vi "NI-Sync_test_case.vi"() -> ()   [LabVIEW 2015]
uses:
  <vilib>/userdefined/High Color/nirio_resource_hc.ctl
  <vilib>/DAQmx/read.llb/DAQmx Read (Analog Wfm 1Chan NSamp).vi
  <instrlib>/niSync/niSync.llb/niSync Initialize (IVI).vi
  <vilib>/DAQmx/create/channels.llb/DAQmx Create Channel (AI-Voltage-Basic).vi
  <vilib>/DAQmx/configure/timing.llb/DAQmx Timing (Sample Clock).vi
  <vilib>/DAQmx/create/channels.llb/DAQmx Create Channel (CO-Pulse Generation-Time).vi
  <vilib>/DAQmx/configure/timing.llb/DAQmx Timing (Implicit).vi
  <vilib>/DAQmx/configure/trigger.llb/DAQmx Start Trigger (Digital Edge).vi
  <vilib>/DAQmx/miscellaneous.llb/DAQmx Fill In Error Info.vi
  <vilib>/FPGAPlugInAG/Dynamic/niLvFpga_Close_Dynamic.vi
  <vilib>/rvi/interface/nirviCloseFPGA/nirviCloseFPGA.xnode
  <resource>/objmgr/daqmx.rc
panel:
  in  "Reset sync cards?":bool
  in  "Pulse delay":dbl=0.0001 format="%#_13g"
  in  "Pulse counter destination terminal":string(combo)="PXI_Star1"
  in  "DAQ pulse gen looking at:":tag="/Timing1/PXI_Star"
  in  "DAQ pulse gen counter":tag="Timing1/ctr2"
  in  "DAQ Physical Channel":tag="DAQ0/ai3"
  in  "Num samples: DAQ":i32=1000
  in  "FPGA AI to plot":i32
  out "RIO":waveform(dbl)(graph)
  out "Interleaved Raw Data":u64[](array[numeric])
  out "Counts":i16[][](array[numeric])
  out "Voltage":dbl[][](array[numeric])
  in  "FPGA delay (x 50ns)":u64=2
  in  "Num samples: RIO":u64=20000
  in  "FPGA name":T1="RIO0" caption="RIO Device"
  out "DAQ":waveform(dbl)(graph)
  in  "DAQ listens to":tag="/DAQ0/PXI_Star"
  in  "DAQ Delay (s)":dbl=1e-07
  in  "RIO Destination Terminal":string(combo)="PXI_Star0"
  in  "DAQ destination terminal":string(combo)="PXI_Star2"
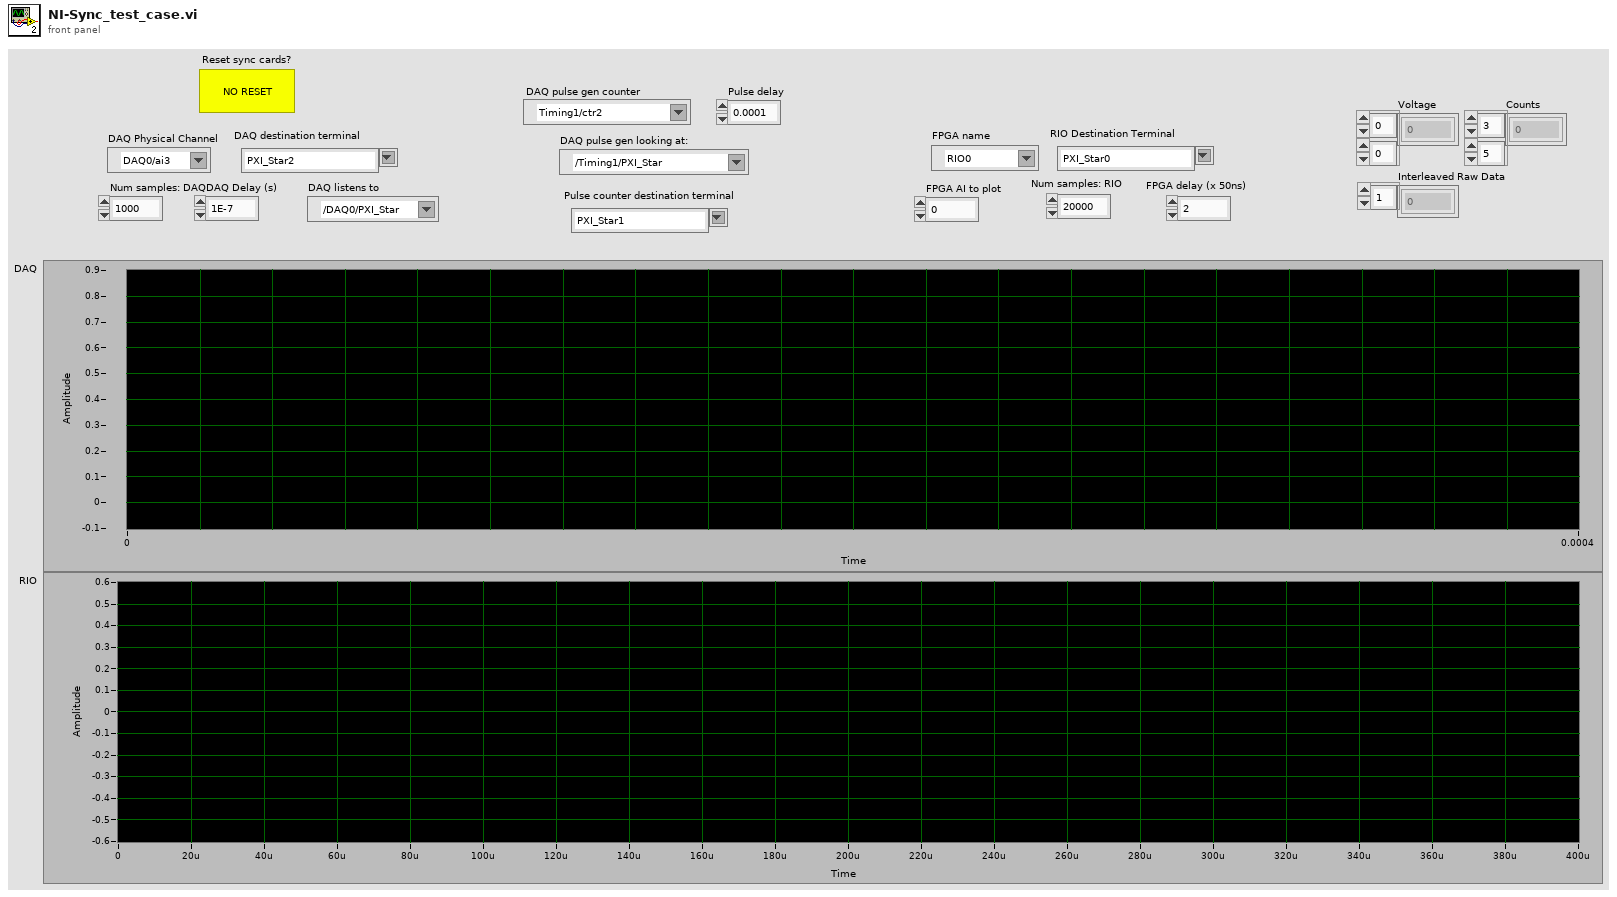
[diagram p1: front panel]
types:
  T1 = typedef "nirio_resource_hc.ctl" = tag
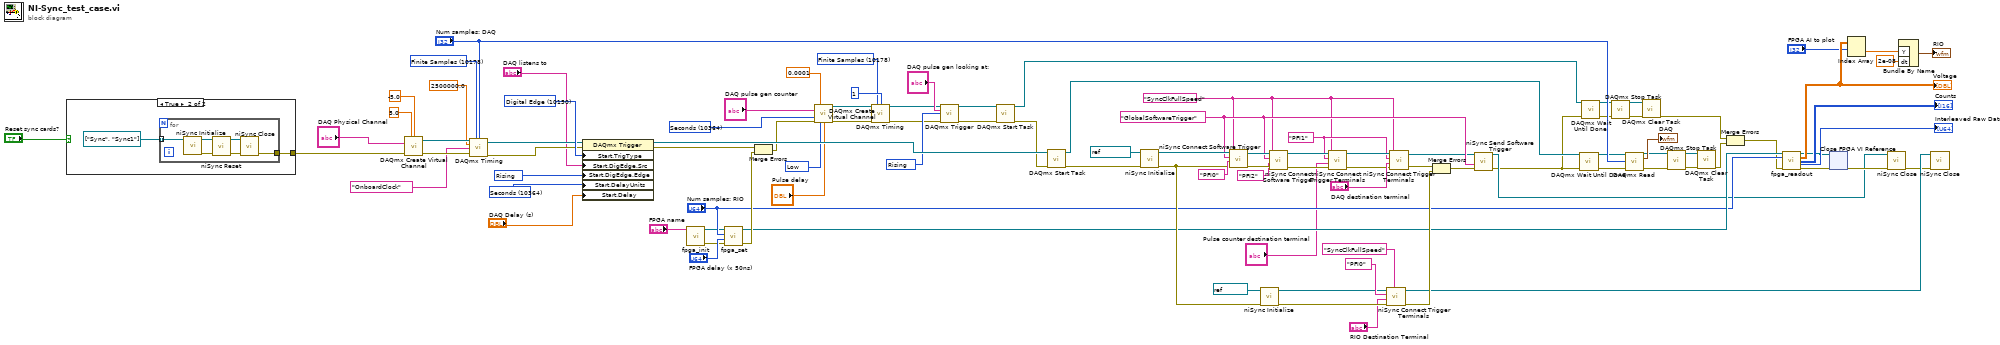
[diagram p0: block diagram]
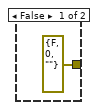
[diagram p2: hidden frame]
diagram:
  w24 = 10178 items=["Finite Samples"=10178, "Continuous Samples"=10123, "Hardware Timed Single Point"=12522] ("sample mode")
  w30 = 10280 items=["Rising"=10280, "Falling"=10171] ("edge")
  w32 = 10364 items=["Seconds"=10364] ("units")
  w33 = 10214 items=["High"=10192, "Low"=10214] ("idle state")
  w66 = 10280 items=["Rising"=10280, "Falling"=10171] ("Start.DigEdge.Edge")
  w71 = 10364 items=["Sample Clock Periods"=10286, "Seconds"=10364, "Ticks"=10304] ("Start.DelayUnits")
  w72 = 10150 items=["Analog Edge"=10099, "Digital Edge"=10150, "Digital Pattern"=10398, "Analog Window"=10103, "None"=10230] ("Start.TrigType")
  w74 = 10178 items=["Finite Samples"=10178, "Continuous Samples"=10123, "Hardware Timed Single Point"=12522] ("sample mode")
  w7 = "PFI1" ("source terminal")
  w6 = "SyncClkFullSpeed" ("synchronization clock")
  w85 = "GlobalSoftwareTrigger" ("source terminal")
  n1 = case shown="True" "Reset sync cards?" {
    tunnel: [errorcluster {"status"=FALSE, "code"=0, "source"=""} ("error out") w103] -> w2
    frame False {
    }
    frame True {
      n2 = for {
        tunnel: refnum<k15>[] ["Sync", "Sync1"] -> [w108] mode=indexing
        tunnel: [w105] -> w103
        n3 = call-poly <instrlib>:"niSync Initialize.vi"("resource name"=w108) -> ("error out"=w109:errorcluster, "instrument handle out"=w110:refnum<k15>)  [unwired: 9 in]
        n4 = call <instrlib>:"niSync Reset.vi"("error in (no error)"=w109, "instrument handle"=w110) -> ("error out"=w106:errorcluster, "instrument handle out"=w107:refnum<k15>)  [unwired: 8 in]
        n5 = call <instrlib>:"niSync Close.vi"("error in (no error)"=w106, "instrument handle"=w107) -> ("error out"=w105:errorcluster)  [unwired: 9 out]
      }
    }
  }
  n6 = call-poly <vilib>:"DAQmx Create Virtual Channel.vi"("maximum value"=5.0, "minimum value"=-5.0, "physical channels"="DAQ Physical Channel", "error in"=w2) -> ("task out"=w78:refnum<k21>, "error out"=w77:errorcluster)  [unwired: 10 in]
  n7 = call-poly <vilib>:"DAQmx Timing.vi"("task/channels in"=w78, "sample mode"=w74, "samples per channel"="Num samples: DAQ", "rate"=2500000.0, "source"=tag "OnboardClock", "error in"=w77) -> ("task out"=w69:refnum<k21>, "error out"=w68:errorcluster)  [unwired: 8 in]
  n8 = property class="DAQmx Trigger"(reference=w69, error in=w68, "Start.TrigType"=w72, "Start.DigEdge.Src"="DAQ listens to", "Start.DigEdge.Edge"=w66, "Start.DelayUnits"=w71, "Start.Delay"="DAQ Delay (s)") -> (reference out=w64:refnum<k21>, error out=w46:errorcluster)
  n9 = call "fpga_init.vi"("FPGA name"="FPGA name") -> ("error out"=w3:errorcluster, "FPGA VI Reference Out"=w4:refnum<k20>)  [unwired: 9 in]
  n10 = call "fpga_set.vi"("error in"=w3, "trigger  delay"="FPGA delay (x 50ns)", "num samples"="Num samples: RIO", "FPGA VI Reference In"=w4) -> ("error out"=w45:errorcluster, "FPGA VI Reference Out"=w43:refnum<k20>)  [unwired: 6 in]
  n11 = Merge Errors(w46, w45) -> (w36:errorcluster)
  n12 = call-poly <vilib>:"DAQmx Create Virtual Channel.vi"("high time"=0.0001, "counter"="DAQ pulse gen counter", "units"=w32, "error in"=w36, "idle state"=w33, "initial delay"="Pulse delay") -> ("task out"=w29:refnum<k21>, "error out"=w27:errorcluster)  [unwired: 8 in]
  n13 = call-poly <vilib>:"DAQmx Timing.vi"("task/channels in"=w29, "sample mode"=w24, "samples per channel"=1, "error in"=w27) -> ("task out"=w28:refnum<k21>, "error out"=w26:errorcluster)  [unwired: 10 in]
  n14 = call-poly <vilib>:"DAQmx Trigger.vi"("task/channels in"=w28, "source"="DAQ pulse gen looking at:", "edge"=w30, "error in"=w26) -> ("task out"=w21:refnum<k21>, "error out"=w23:errorcluster)  [unwired: 10 in]
  n15 = call <vilib>:"DAQmx Start Task.vi"("task/channels in"=w21, "error in"=w23) -> ("task out"=w16:refnum<k21>, "error out"=w22:errorcluster)  [unwired: 12 in]
  n16 = call <vilib>:"DAQmx Start Task.vi"("task/channels in"=w64, "error in"=w22) -> ("task out"=w39:refnum<k21>, "error out"=w65:errorcluster)  [unwired: 12 in]
  n17 = call-poly <instrlib>:"niSync Initialize.vi"("error in (no error)"=w65, "resource name"=refnum<k15> "Sync") -> ("error out"=w73:errorcluster, "instrument handle out"=w99:refnum<k15>)  [unwired: 1 in, 7 out]
  n18 = call <instrlib>:"niSync Connect Software Trigger.vi"("synchronization clock"=w6, "error in (no error)"=w73, "destination terminal"="PFI0", "source terminal"=w85, "instrument handle"=w99) -> ("error out"=w96:errorcluster, "instrument handle out"=w97:refnum<k15>)  [unwired: 2 in, 3 out]
  n19 = call-poly <instrlib>:"niSync Initialize.vi"("error in (no error)"=w73, "resource name"=refnum<k15> "Sync1") -> ("error out"=w94:errorcluster, "instrument handle out"=w90:refnum<k15>)  [unwired: 1 in, 7 out]
  n20 = call <instrlib>:"niSync Connect Software Trigger.vi"("synchronization clock"=w6, "error in (no error)"=w96, "destination terminal"="PFI2", "source terminal"=w85, "instrument handle"=w97) -> ("error out"=w9:errorcluster, "instrument handle out"=w11:refnum<k15>)  [unwired: 2 in, 3 out]
  n21 = call <instrlib>:"niSync Connect Trigger Terminals.vi"("synchronization clock"=w6, "error in (no error)"=w9, "destination terminal"="Pulse counter destination terminal", "source terminal"=w7, "instrument handle"=w11) -> ("error out"=w8:errorcluster, "instrument handle out"=w10:refnum<k15>)  [unwired: 5 in]
  n22 = call <instrlib>:"niSync Connect Trigger Terminals.vi"("synchronization clock"="SyncClkFullSpeed", "error in (no error)"=w94, "destination terminal"="RIO Destination Terminal", "source terminal"="PFI0", "instrument handle"=w90) -> ("error out"=w91:errorcluster, "instrument handle out"=w83:refnum<k15>)  [unwired: 5 in]
  n23 = call <instrlib>:"niSync Connect Trigger Terminals.vi"("synchronization clock"=w6, "error in (no error)"=w8, "destination terminal"="DAQ destination terminal", "source terminal"=w7, "instrument handle"=w10) -> ("error out"=w89:errorcluster, "instrument handle out"=w84:refnum<k15>)  [unwired: 5 in]
  n24 = Merge Errors(w89, w91) -> (w86:errorcluster)
  n25 = call <instrlib>:"niSync Send Software Trigger.vi"("error in (no error)"=w86, "source terminal"=w85, "instrument handle"=w84) -> ("error out"=w15:errorcluster, "instrument handle out"=w41:refnum<k15>)  [unwired: 7 out]
  n26 = call <vilib>:"DAQmx Wait Until Done.vi"("task/channels in"=w39, "error in"=w15) -> ("task out"=w40:refnum<k21>, "error out"=w38:errorcluster)  [unwired: 12 in]
  n27 = call <vilib>:"DAQmx Wait Until Done.vi"("task/channels in"=w16, "error in"=w15) -> ("task out"=w18:refnum<k21>, "error out"=w17:errorcluster)  [unwired: 12 in]
  n28 = call <vilib>:"DAQmx Stop Task.vi"("task/channels in"=w18, "error in"=w17) -> ("task out"=w19:refnum<k21>, "error out"=w20:errorcluster)  [unwired: 12 in]
  n29 = call-poly <vilib>:"DAQmx Read.vi"("task/channels in"=w40, "number of samples per channel"="Num samples: DAQ", "error in"=w38) -> ("task out"=w61:refnum<k21>, "data"=→"DAQ":waveform(dbl), "error out"=w62:errorcluster)  [unwired: 10 in]
  n30 = call <vilib>:"DAQmx Clear Task.vi"("task in"=w19, "error in"=w20) -> ("error out"=w14:errorcluster)  [unwired: 13 in]
  n31 = call <vilib>:"DAQmx Stop Task.vi"("task/channels in"=w61, "error in"=w62) -> ("task out"=w59:refnum<k21>, "error out"=w58:errorcluster)  [unwired: 12 in]
  n32 = call <vilib>:"DAQmx Clear Task.vi"("task in"=w59, "error in"=w58) -> ("error out"=w13:errorcluster)  [unwired: 13 in]
  n33 = Merge Errors(w14, w13) -> (w12:errorcluster)
  n34 = call "fpga_readout.vi"("FPGA VI Reference In"=w43, "samples"="Num samples: RIO", "error in"=w12) -> ("FPGA Reference Out"=w44:refnum<k20>, "Voltage"=w49:dbl[][], "Counts"=→"Counts":i16[][], "Interleaved Raw Data"=→"Interleaved Raw Data":u64[], "error out"=w55:errorcluster)  [unwired: 8 in]
  "Voltage" <- w49
  n35 = xnode "Close FPGA VI Reference"("FPGA VI Reference In"=w44, "error in"=w55) -> ("error out"=w47:errorcluster)
  n36 = Index Array(array=w49, index (row)="FPGA AI to plot") -> (element=w53:dbl[])  [unwired: 1 in]
  n37 = call <instrlib>:"niSync Close.vi"("error in (no error)"=w47, "instrument handle"=w41) -> ("error out"=w82:errorcluster)  [unwired: 9 out]
  n38 = Bundle By Name("Y"=w53, "dt"=2e-08) -> (→"RIO":waveform(dbl))  [unwired: 1 in]
  n39 = call <instrlib>:"niSync Close.vi"("error in (no error)"=w82, "instrument handle"=w83) -> ()  [unwired: 10 out]
